vi "RSZVB Configure Chopped Pulse Profile.vi"(7 "Delay Increment (0.0 s)":dbl format="%^.3e", 8 "error in (no error)":errorcluster {"code" format="%.0x"}, 9 "Chopped Pulse Profile Mode (Off)":bool, 10 "Channel (1)":i32=1, 11 "VISA session":refnum<visa-resource-name>) -> (0 "error out":errorcluster {"code" format="%.0x"}, 3 "dup VISA session":refnum<visa-resource-name>)   [LabVIEW 2011]
doc: "This VI defines the properties of the chopped pulse profile.\n\nNote(s):\n\n(1) This VI is available only with option R&S ZVA-K27.\n\nRemote-control command(s):\n[SENSe<Ch>:]PULSe:GENerator<gen_no>:CPPRofile\n[SENSe<Ch>:]PULSe:GENerator<gen_no>:DINCrement"
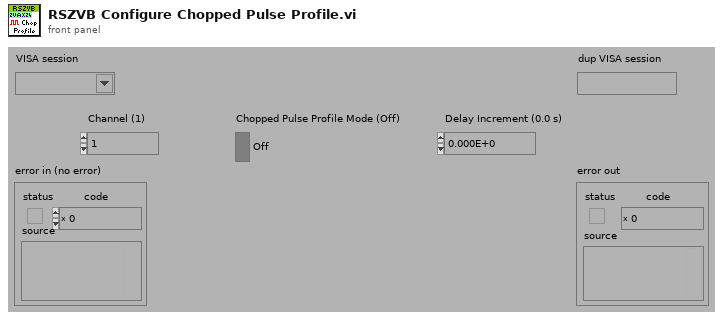
[diagram p1: front panel]
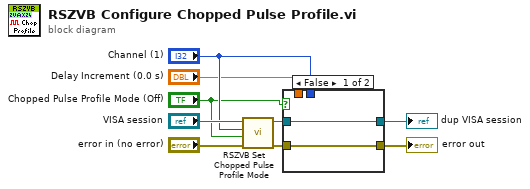
[diagram p0: block diagram]
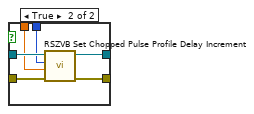
[diagram p2: hidden frame]
diagram:
  n1 = call "RSZVB Set Chopped Pulse Profile Mode.vi"("error in (no error)"="error in (no error)", "Chopped Pulse Profile Mode (Off)"="Chopped Pulse Profile Mode (Off)", "Channel (1)"="Channel (1)", "VISA session"="VISA session") -> ("error out"=w6:errorcluster, "dup VISA session"=w7:refnum<visa-resource-name>)  [unwired: 6 in]
  n2 = case shown="False" "Chopped Pulse Profile Mode (Off)" {
    tunnel: w7 -> [w11 w17]
    tunnel: w6 -> [w10 w16]
    tunnel: [w10 w15] -> w5
    tunnel: [w11 w14] -> w4
    tunnel: "Channel (1)" -> [_ w13]
    tunnel: "Delay Increment (0.0 s)" -> [_ w12]
    frame False {
    }
    frame True {
      n3 = call "RSZVB Set Chopped Pulse Profile Delay Increment.vi"("error in (no error)"=w16, "Delay Increment (0.0 s)"=w12, "Channel (1)"=w13, "VISA session"=w17) -> ("error out"=w15:errorcluster, "dup VISA session"=w14:refnum<visa-resource-name>)  [unwired: 6 in]
    }
  }
  "error out" <- w5
  "dup VISA session" <- w4
